vi "Set Manifold All Channels.vi"(8 "error in":errorcluster, 9 "On/Off":bool, 11 "Gantry in":refnum<class "Gantry Class.lvclass">) -> (0 "error out":errorcluster, 3 "Gantry out":refnum<class "Gantry Class.lvclass">)   [LabVIEW 2017, in "Gantry Class.lvclass"]
uses:
  Gantry Class.lvclass
  Gantry Class.lvclass/Gantry Class.ctl
  <vilib>/DAQmx/write.llb/DAQmx Write (Digital 1D Bool 1Chan 1Samp).vi
  <vilib>/DAQmx/miscellaneous.llb/DAQmx Fill In Error Info.vi
  WorkTable Class/WorkTable Class.lvclass
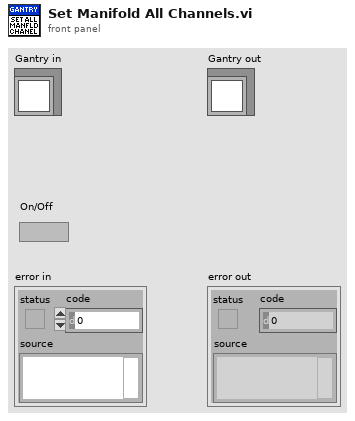
[diagram p1: front panel]
types:
  T1 = typedef "Worktable_Manifold.ctl" = cluster{"Vacuum Channel Status":T2[], "Vacuum Channel Names":T3[]}
  T2 = typedef "Worktable_Manifold Channel.ctl" = cluster{"Enabled":bool, "Hardware Path":string}
  T3 = typedef "Worktable_Manifold Channel Names.ctl" = cluster{"Channel Name":string, "Channel Number":i8}
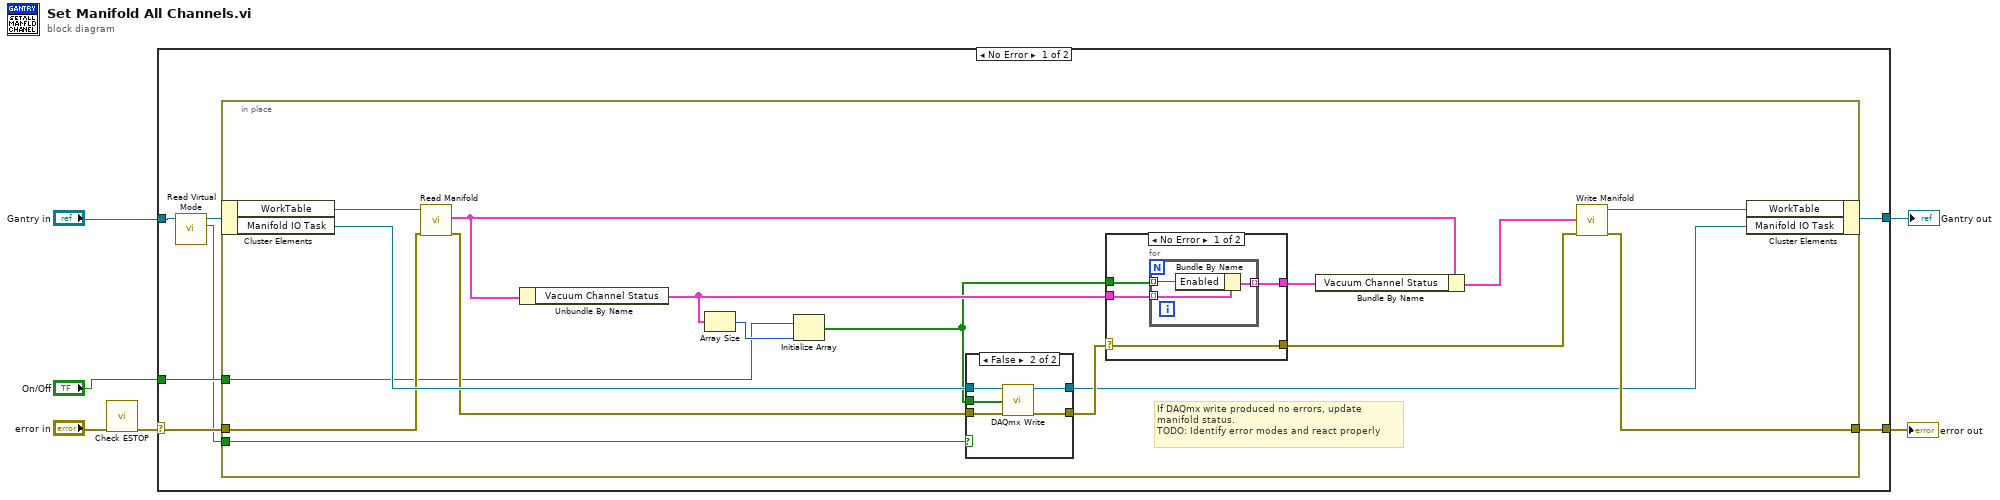
[diagram p0: block diagram]
diagram:
  n1 = call "Check ESTOP.vi"("error in"="error in") -> ("error out"=w2:errorcluster)  [unwired: 10 in]
  n2 = case shown="No Error" w2 {
    selector: w2 -> [w12 w48]
    tunnel: [w10 w48] -> w6
    tunnel: [w11 w47] -> w5
    tunnel: "Gantry in" -> [w9 w47]
    tunnel: "On/Off" -> [w13 _]
    frame No Error {
      n3 = call-dynamic "Read Virtual Mode.vi"("Gantry Class in"=w9) -> ("Virtual Mode"=w7:bool, "Gantry Class out"=w8:refnum<class "Gantry Class.lvclass">)  [unwired: 8 in, 1 out]
      n4 = in-place {
        in-place-border: w13 -> [w15]
        in-place-border: w12 -> [w23]
        in-place-border: [w28] -> w10
        in-place-border: w7 -> [w20]
        # "If DAQmx write produced no errors, update \nmanifold status.\nTODO: Identify error modes and react properly"
        n5 = in-place-cluster #1(w8) -> ("WorkTable"=w26:refnum<class "WorkTable Class.lvclass">, "Manifold IO Task"=w24:refnum<k21>)
        n6 = call-dynamic "Read Manifold.vi"("error in (no error)"=w23, "WorkTable Class in"=w26) -> ("error out"=w22:errorcluster, "Manifold"=w19:T1)  [unwired: 7 in, 1 out]
        n7 = Unbundle By Name(w19) -> ("Vacuum Channel Status"=w17:T2[])
        n8 = Array Size(array=w17) -> (size(s)=w16:i32)
        n9 = Initialize Array(w15, w16) -> (w14:bool[])
        n10 = case shown="False" w20 {
          tunnel: [w32 w37] -> w30
          tunnel: w14 -> [_ w36]
          tunnel: w24 -> [w31 w35]
          tunnel: w22 -> [w32 w34]
          tunnel: [w31 w33] -> w21
          frame True {
          }
          frame False {
            n11 = call-poly <vilib>:"DAQmx Write.vi"("task/channels in"=w35, "data"=w36, "error in"=w34) -> ("task out"=w33:refnum<k21>, "error out"=w37:errorcluster)  [unwired: 10 in, 1 out]
          }
        }
        n12 = case shown="No Error" w30 {
          selector: w30 -> [w38 w46]
          tunnel: w14 -> [w40 _]
          tunnel: w17 -> [w41 w45]
          tunnel: [w38 w46] -> w29
          tunnel: [w39 w45] -> w27
          frame No Error {
            n13 = for {
              tunnel: w41 -> [w44] mode=indexing
              tunnel: w40 -> [w43] mode=indexing
              tunnel: [w42] -> w39 mode=indexing
              n14 = Bundle By Name(cluster=w44, "Enabled"=w43) -> (w42:T2)
            }
          }
          frame Error {
          }
        }
        n15 = Bundle By Name(cluster=w19, "Vacuum Channel Status"=w27) -> (w18:T1)
        n16 = call "Write Manifold.vi"("error in (no error)"=w29, "Manifold"=w18) -> ("error out"=w28:errorcluster, "WorkTable Class out"=w25:refnum<class "WorkTable Class.lvclass">)  [unwired: 8 in]
        n17 = in-place-cluster #1("WorkTable"=w25, "Manifold IO Task"=w21) -> (w11:refnum<class "Gantry Class.lvclass">)
      }
    }
    frame Error {
    }
  }
  "error out" <- w6
  "Gantry out" <- w5
